vi "Strip N Paths.vi"(9 "N":i32, 11 "path":path) -> (1 "[Stripped]":string[](array[string]), 3 "stripped path":path)   [LabVIEW 2013, in "FileIO lib.lvlib"]
uses:
  FileIO lib.lvlib
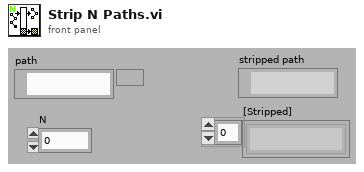
[diagram p1: front panel]
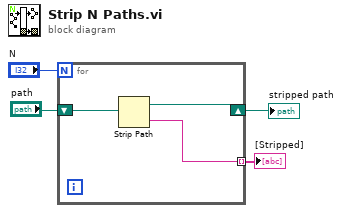
[diagram p0: block diagram]
diagram:
  n1 = for {
    N: "N" -> [_]
    shift-right: [w6] -> w3
    shift-left: "path" -> [w7]
    tunnel: [w5] -> w1 mode=indexing
    n2 = Strip Path(path=w7) -> (stripped path=w6:path, name=w5:string)
  }
  "stripped path" <- w3
  "[Stripped]" <- w1
